vi "Moving.vi"(6 "number of samples":i32, 9 "rate":dbl, 10 "Velocity value (mm/s)":dbl, 11 "VISA Refnum in":refnum<visa-resource-name>) -> (0 "error out":errorcluster, 1 "Displacement":dbl, 2 "Total time":dbl, 3 "VISA Refnum out":refnum<visa-resource-name>, 5 "Axis out":i32=1)   [LabVIEW 2021]
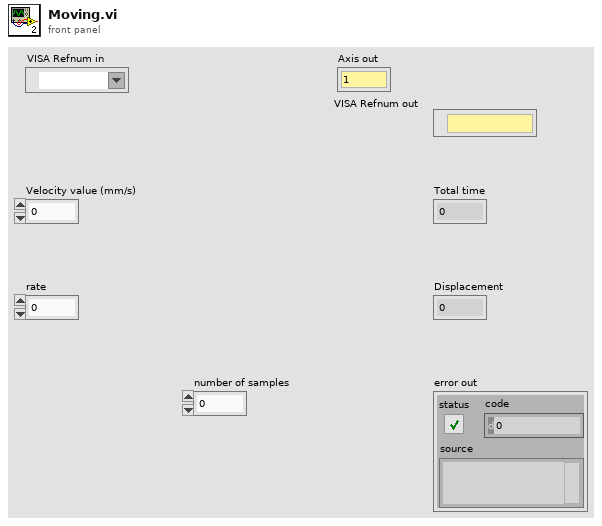
[diagram p1: front panel]
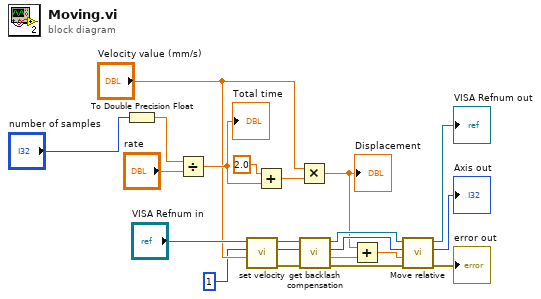
[diagram p0: block diagram]
diagram:
  n1 = To Double Precision Float(number="number of samples") -> (double precision float=w9:dbl)
  n2 = Divide(x=w9, y="rate") -> (x/y=w6:dbl)
  "Total time" <- w6
  n3 = call <userlib>:"set velocity.vi"("Velocity value (units/s)"="Velocity value (mm/s)", "Axis in"=1, "VISA Handle in"="VISA Refnum in") -> ("error out"=w11:errorcluster, "Axis out"=w12:i32, "VISA Handle out"=w13:refnum<visa-resource-name>)  [unwired: 3 in, 1 out]
  n4 = Add(x=2.0, y=w6) -> (x+y=w7:dbl)
  n5 = Multiply(x="Velocity value (mm/s)", y=w7) -> (x*y=w14:dbl)
  "Displacement" <- w14
  n6 = call <userlib>:"get backlash compensation.vi"("error in"=w11, "Axis in"=w12, "VISA Handle in"=w13) -> ("error out"=w19:errorcluster, "Backlash compensation value (units)"=w15:dbl, "Axis out"=w18:i32, "VISA Handle out"=w17:refnum<visa-resource-name>)  [unwired: 2 in, 1 out]
  n7 = Add(x=w14, y=w15) -> (x+y=w16:dbl)
  n8 = call <userlib>:"Move relative.vi"("error in"=w19, "Displacement (units)"=w16, "Axis in"=w18, "VISA Handle in"=w17) -> ("error out"=→"error out":errorcluster, "Axis out"=→"Axis out":i32, "VISA Handle out"=→"VISA Refnum out":refnum<visa-resource-name>)  [unwired: 2 in, 1 out]
